vi "FTW-ProjectManager-Construct.vi"(5 "Project Reference":refnum<vi>, 11 "error in":errorcluster) -> (4 "Project Manager":refnum<class "FTW-ProjectManager.lvclass">, 6 "Project Name":string, 15 "error out":errorcluster)   [LabVIEW 2012, in "FTW-ProjectManager.lvclass"]
uses:
  FTW-ProjectManager.lvclass
  FTW-ProjectManager.lvclass/FTW-ProjectManager.ctl
panel:
  # "Inputs"
  # "Outputs"
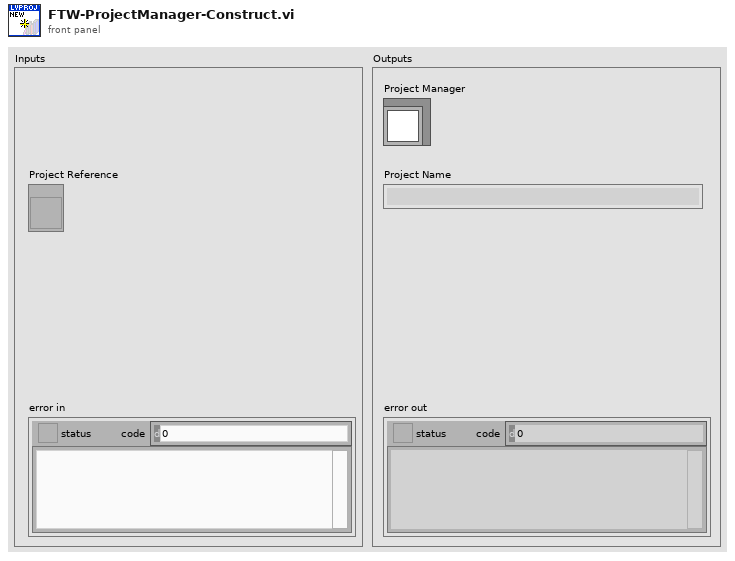
[diagram p1: front panel]
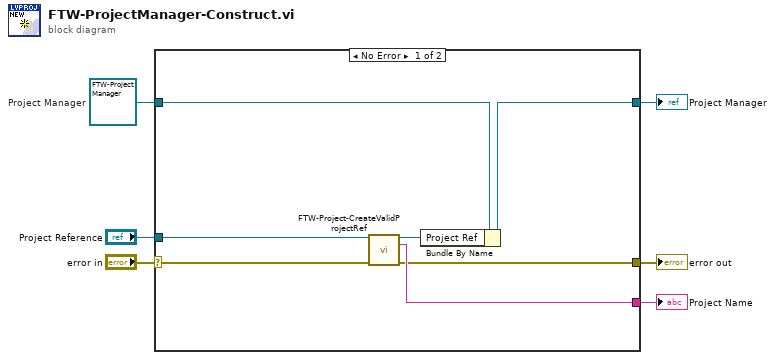
[diagram p0: block diagram]
diagram:
  w5 = refnum<class "FTW-ProjectManager.lvclass"> refnum  # Project Manager
  n1 = case shown="No Error" "error in" {
    selector: "error in" -> [w7 w15]
    tunnel: [w8 w15] -> w6
    tunnel: [w12 w14] -> w4
    tunnel: w5 -> [w13 w14]
    tunnel: "Project Reference" -> [w11 _]
    tunnel: [w9 _] -> w1
    frame No Error {
      n2 = call "FTW-Project-CreateValidProjectRef.vi"("Project Ref (blank for Active Project)"=w11, "error in"=w7) -> ("Project Ref"=w10:refnum<vi>, "Name"=w9:string, "error out"=w8:errorcluster)  [unwired: 11 in]
      n3 = Bundle By Name(cluster=w13, "Project Ref"=w10) -> (w12:refnum<class "FTW-ProjectManager.lvclass">)
    }
    frame Error {
    }
  }
  "error out" <- w6
  "Project Manager" <- w4
  "Project Name" <- w1
